vi "Pop.vi"(8 "error in (no error)":errorcluster, 11 "UPNCalculator in":refnum<class "UPNCalculator.lvclass">) -> (0 "error out":errorcluster, 2 "Element":dbl, 3 "UPNCalculator out":refnum<class "UPNCalculator.lvclass">)   [LabVIEW 2012, in "UPNCalculator Actor.lvlib" / "UPNCalculator.lvclass"]
doc: "Pop an element from top of stack."
uses:
  UPNCalculator.lvclass
  UPNCalculator.lvclass/UPNCalculator.ctl
  Stack/Stack.lvclass
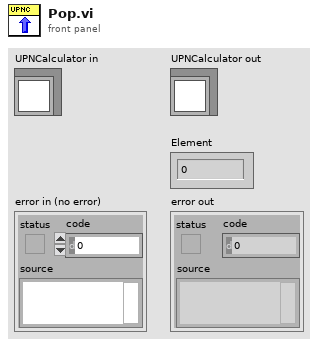
[diagram p1: front panel]
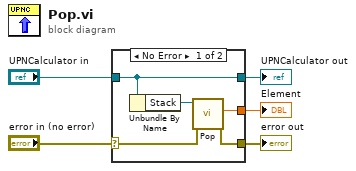
[diagram p0: block diagram]
diagram:
  n1 = case shown="No Error" "error in (no error)" {
    selector: "error in (no error)" -> [w8 w12]
    tunnel: [w7 w12] -> w4
    tunnel: [w10 w11] -> w2
    tunnel: "UPNCalculator in" -> [w10 w11]
    tunnel: [w6 _] -> w1
    frame No Error {
      n2 = Unbundle By Name(w10) -> ("Stack"=w9:refnum<class "Stack.lvclass">)
      n3 = call "Pop.vi"("error in (no error)"=w8, "Stack in"=w9) -> ("error out"=w7:errorcluster, "Element"=w6:dbl)  [unwired: 7 in, 1 out]
    }
    frame Error {
    }
  }
  "error out" <- w4
  "UPNCalculator out" <- w2
  "Element" <- w1
